vi "rms 2.vi"() -> ()   [LabVIEW 2017]
panel:
  out "Numeric":dbl
  in  "String":string
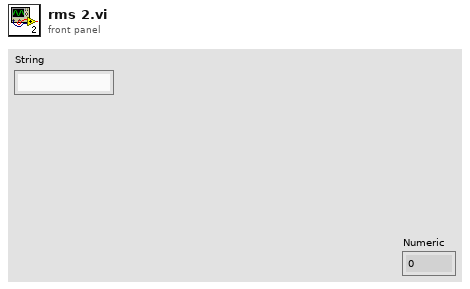
[diagram p1: front panel]
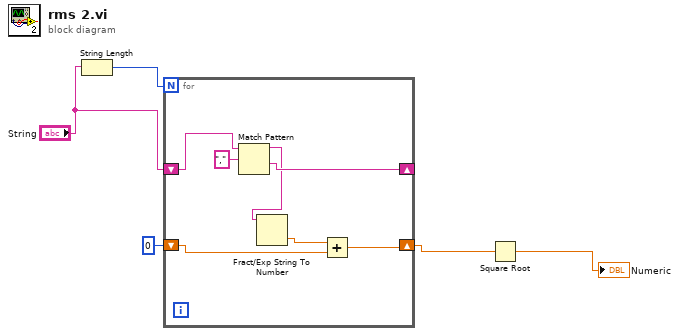
[diagram p0: block diagram]
diagram:
  n1 = String Length(string="String") -> (length=w5:i32)
  n2 = for {
    N: w5 -> [_]
    shift-right: [w11] -> _
    shift-left: "String" -> [w10]
    shift-right: [w8] -> w2
    shift-left: 0 -> [w7]
    n3 = Match Pattern(string=w10, regular expression="," ("search string/char (-)")) -> (before substring=w6:string, after substring=w11:string)  [unwired: 1 in, 2 out]
    n4 = Fract/Exp String To Number(string=w6) -> (number=w9:dbl)  [unwired: 3 in, 1 out]
    n5 = Add(x=w9, y=w7) -> (x+y=w8:dbl)
  }
  n6 = Square Root(x=w2) -> (sqrt(x)=→"Numeric":dbl)
